vi "Actor Core.vi"(8 "error in":errorcluster, 11 "CS++DCPwrGui.lvclass":refnum<class "CS++DCPwrGui.lvclass">) -> (0 "error out":errorcluster, 3 "Actor out":refnum<class "Actor.lvclass">)   [LabVIEW 2013, in "CS++DCPwrGui.lvlib" / "CS++DCPwrGui.lvclass"]
doc: "(<B>Filename</B>: Actor Framework.lvlib:Actor.lvclass:Actor Core.vi)\n\nReceives messages to the actor, reacts to them, and initiates any error handling that may shut the actor down.\n\nDescendant classes may override this VI to append parallel tasks for the actor to complete while it handles messages. Overrides use the Call Parent Method node."
uses:
  CS++DCPwrGui.lvclass
  <vilib>/ActorFramework/Actor/Actor.lvclass
  Core/Classes/CS++ProcessVariables/ProcessVariable/PV.lvclass
  Core/Actors/CS++SVMonitor/CS++SVMonitor.lvclass
  Core/Actors/CS++BaseActor/CS++BaseActor.lvclass/CS++BaseActor.ctl
  <vilib>/ActorFramework/Actor/Actor.lvclass/Actor.ctl
  <vilib>/ActorFramework/Message Enqueuer/Message Enqueuer.lvclass/Message Enqueuer.ctl
  Core/Actors/CS++DeviceGUIActor/CS++DeviceGUIActor.lvclass/CS++DeviceGUIActor.ctl
  Core/Classes/CS++BaseClasses/Factory/CS++Factory.lvclass
  Core/Actors/CS++PVMonitor/CS++PVMonitor.lvclass/CS++PVMonitor.ctl
  Core/Actors/CS++GUIActor/CS++GUIActor.lvclass/CS++GUIActor.ctl
  CS++DMMGui Messages/UpdatePV/UpdatePV.lvclass
  Core/Actors/CS++PVMonitor Messages/Register PVs Msg/Register PVs Msg.lvclass/Register PVs Msg.ctl
  CS++DCPwrGui.lvclass/CS++DCPwrGui.ctl
  Core/Actors/CS++DeviceGUIActor/CS++DeviceGUIActor.lvclass
  Core/Classes/CS++ProcessVariables/ProcessVariable/PV.lvclass/PV.ctl
  Core/Actors/CS++DeviceGUIActor/Read Resource Name.vi
  Core/Actors/CS++DeviceGUIActor/Read Driver Revision.vi
  Core/Actors/CS++DeviceGUIActor/Read Firmware Revision.vi
  Core/Actors/CS++DeviceGUIActor/Read Self-Test Result Code.vi
  Core/Actors/CS++DeviceGUIActor/Read Self-Test Result Message.vi
  Core/Classes/CS++ProcessVariables/ProcessVariable/Read Data.vi
  <vilib>/ActorFramework/Message Enqueuer/Init from Existing Queue.vi
  <vilib>/ActorFramework/Message Enqueuer/Enqueue.vi
  <vilib>/ActorFramework/Message Priority Queue/Priority Enqueue.vi
  <vilib>/ActorFramework/Message Enqueuer/Message Enqueuer.lvclass
  Core/Actors/CS++PVMonitor Messages/Register PVs Msg/Register PVs Msg.lvclass
  <vilib>/ActorFramework/Stop Msg/Stop Msg.lvclass
  Core/Actors/CS++BaseActor/CS++BaseActor.lvclass
  Core/Actors/CS++GUIActor/CS++GUIActor.lvclass
  Core/Actors/CS++PVMonitor/CS++PVMonitor.lvclass
panel:
  in  "Tab Control":enum32{"Info", "Configuration"}(tab)
  out "Actor Name":string
  out "Driver Revision":string
  out "Firmware Revision":string
  out "Self-Test Result Code":i32
  out "Self-Test Result Message":string
  out "Resource Name":string
  in  "Configuration Tab":enum32{"General", "Trigger"}(tab)
  in  "Stop Button":bool
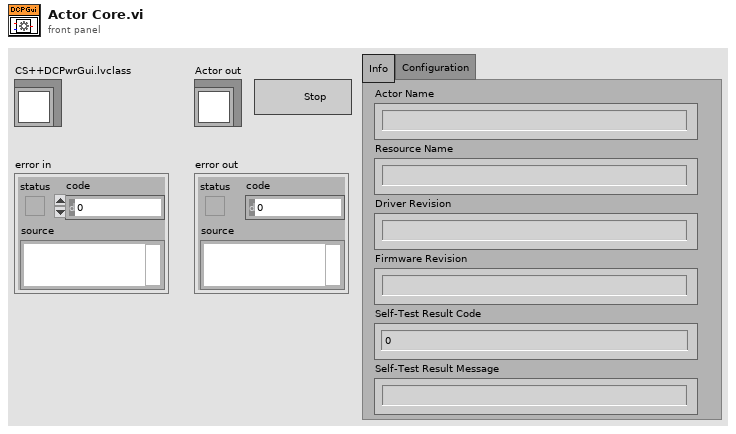
[diagram p1: front panel]
types:
  T1 = enum32{"Invalid", "Standard", "Closed", "Hidden", "Minimized", "Maximized"}
  T2 = cluster{string, "CS++DMMGui.lvlib:UpdatePV.lvclass":refnum<class "UpdatePV.lvclass">}
  T3 = cluster{"Self Enqueuer":refnum<class "Message Enqueuer.lvclass">, cluster{string, "CS++DMMGui.lvlib:UpdatePV.lvclass":refnum<class "UpdatePV.lvclass">}[]}
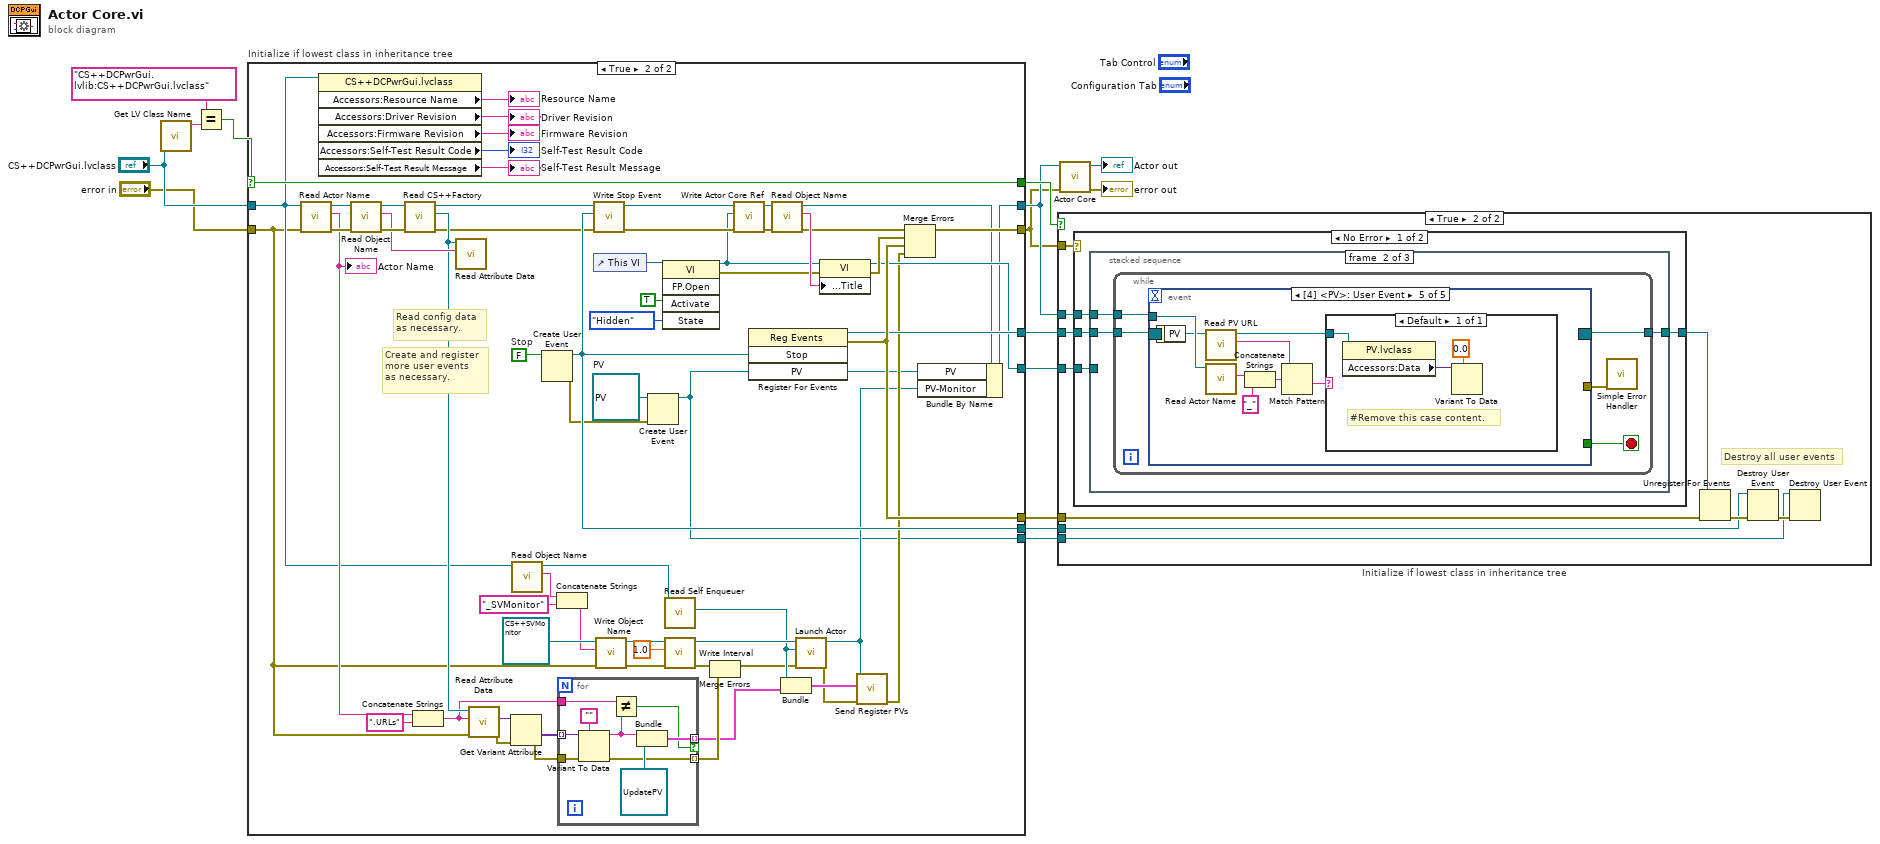
[diagram p0: block diagram]
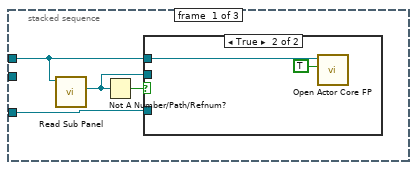
[diagram p4: hidden frame]
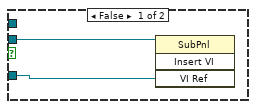
[diagram p5: hidden frame]
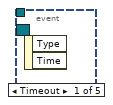
[diagram p6: hidden frame]
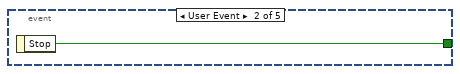
[diagram p7: hidden frame]
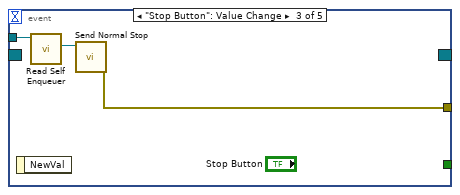
[diagram p8: hidden frame]
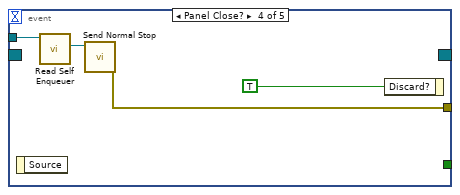
[diagram p9: hidden frame]
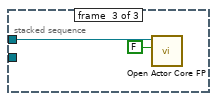
[diagram p10: hidden frame]
diagram:
  n1 = call <vilib>:"Get LV Class Name.vi"("object"="CS++DCPwrGui.lvclass") -> ("class name"=w13:string)  [unwired: 9 in, 1 out]
  n2 = Equal?(x="CS++DCPwrGui.lvlib:CS++DCPwrGui.lvclass" ("class name"), y=w13) -> (x = y?=w7:bool)
  n3 = case "Initialize if lowest class in inheritance tree" shown="True" w7 {
    selector: w7 -> [w16 w58]
    tunnel: [w17 w82] -> w2
    tunnel: "error in" -> [w17 w44]
    tunnel: [w18 w48] -> w3
    tunnel: "CS++DCPwrGui.lvclass" -> [w18 w47]
    tunnel: [_ w75] -> w11
    tunnel: [_ w74] -> w10
    tunnel: [_ w50] -> w9
    tunnel: [_ w65] -> w8
    tunnel: [w16 w58] -> w6
    tunnel: [_ w43] -> w1
    frame False {
    }
    frame True {
      w42 = refnum<class "PV.lvclass"> refnum  # PV
      w77 = FALSE  # Stop
      # "Create and register \nmore user events\nas necessary."
      # "Read config data\nas necessary."
      n4 = call "Read Actor Name.vi"("error in (no error)"=w44, "CS++GUIActor in"=w47) -> ("error out"=w68:errorcluster, "Actor Name"=w66:string, "CS++GUIActor out"=w69:refnum<class "CS++DCPwrGui.lvclass">)  [unwired: 7 in]
      "Actor Name" <- w66
      n5 = property class="CS++DCPwrGui.lvclass"(reference=w47) -> ("Accessors:Resource Name"=→"Resource Name":string, "Accessors:Driver Revision"=→"Driver Revision":string, "Accessors:Firmware Revision"=→"Firmware Revision":string, "Accessors:Self-Test Result Code"=→"Self-Test Result Code":i32, "Accessors:Self-Test Result Message"=→"Self-Test Result Message":string)  [unwired: 1 in, 2 out]
      n6 = call "Read Object Name.vi"("error in (no error)"=w68, "CS++BaseActor in"=w69) -> ("error out"=w71:errorcluster, "Object Name"=w70:string, "CS++BaseActor out"=w72:refnum<class "CS++DCPwrGui.lvclass">)  [unwired: 7 in]
      n7 = call "Read CS++Factory.vi"("error in (no error)"=w71, "CS++BaseActor in"=w72) -> ("error out"=w64:errorcluster, "CS++Factory"=w67:refnum<class "CS++Factory.lvclass">, "CS++BaseActor out"=w57:refnum<class "CS++DCPwrGui.lvclass">)  [unwired: 7 in]
      n8 = Concatenate Strings(w66, ".URLs" ("string")) -> (w23:string)
      n9 = call-dynamic "Read Attribute Data.vi"("Object Name"=w70, "CS++Factory in"=w67) -> ()  [unwired: 7 in, 3 out]
      n10 = call-dynamic "Read Attribute Data.vi"("error in (no error)"=w44, "Object Name"=w23, "CS++Factory in"=w67) -> ("error out"=w24:errorcluster, "Attribute Data"=w25:variant)  [unwired: 6 in, 1 out]
      n11 = Get Variant Attribute(Variant=w25, error in=w24) -> (values=w26:variant[], error out=w27:errorcluster)  [unwired: 2 in, 2 out]
      n12 = call "Read Object Name.vi"("CS++BaseActor in"=w47) -> ("Object Name"=w33:string, "CS++BaseActor out"=w32:refnum<class "CS++DCPwrGui.lvclass">)  [unwired: 8 in, 1 out]
      n13 = Create User Event(user event datatype=w77) -> (user event=w65:refnum<user-event>, error out=w41:errorcluster)  [unwired: 1 in]
      n14 = Concatenate Strings(w33, "_SVMonitor" ("Object Name")) -> (w37:string)
      n15 = for {
        tunnel: [w91] -> w19 mode=indexing if=w87
        tunnel: w26 -> [w90] mode=indexing
        tunnel: w27 -> [w89]
        tunnel: w23 -> [w88]
        tunnel: [w83] -> w20 mode=indexing
        n16 = Variant To Data(error in=w89, type="", Variant=w90) -> (data=w84:string, error out=w83:errorcluster)
        n17 = Not Equal?(x=w88, y=w84) -> (x != y?=w87:bool)
        n18 = Bundle(w84, "CS++DMMGui.lvlib:UpdatePV.lvclass"=refnum<class "UpdatePV.lvclass"> refnum) -> (w91:T2)  [unwired: 1 in]
      }
      n19 = call "Write Stop Event.vi"("error in (no error)"=w64, "Stop"=w65, "CS++GUIActor in"=w57) -> ("error out"=w62:errorcluster, "CS++GUIActor out"=w63:refnum<class "CS++DCPwrGui.lvclass">)  [unwired: 7 in]
      n20 = control-ref of="This VI"() -> (w81:refnum<vi>)
      n21 = call "Write Object Name.vi"("error in (no error)"=w44, "Object Name"=w37, "CS++BaseActor in"=refnum<class "CS++SVMonitor.lvclass"> refnum ("CS++SVMonitor.lvlib:CS++SVMonitor.lvclass")) -> ("error out"=w40:errorcluster, "CS++BaseActor out"=w38:refnum<class "CS++SVMonitor.lvclass">)  [unwired: 7 in]
      n22 = Create User Event(user event datatype=w42, error in=w41) -> (user event=w43:refnum<user-event>)  [unwired: 1 out]
      n23 = invoke class="VI" method="FP.Open"(reference=w81, "Activate"=TRUE ("Activate?"), "State"=T1."Hidden") -> (reference out=w51:refnum<vi>, error out=w73:errorcluster)  [unwired: 2 in, 3 out]
      n24 = call <vilib>:"Read Self Enqueuer.vi"("Actor"=w32) -> ("Self Enqueuer"=w31:refnum<class "Message Enqueuer.lvclass">)  [unwired: 10 in]
      n25 = call "Write Interval.vi"("error in (no error)"=w40, "Interval"=dbl[unit] 1.0, "CS++PVMonitor in"=w38) -> ("error out"=w22:errorcluster, "CS++PVMonitor out"=w36:refnum<class "CS++SVMonitor.lvclass">)  [unwired: 7 in]
      n26 = Merge Errors(w22, w20) -> (w21:errorcluster)
      n27 = call "Write Actor Core Ref.vi"("error in (no error)"=w62, "Actor Core Ref"=w51, "CS++BaseActor in"=w63) -> ("error out"=w61:errorcluster, "CS++BaseActor out"=w60:refnum<class "CS++DCPwrGui.lvclass">)  [unwired: 7 in]
      n28 = register-events(w65, w43) -> (reference out=w74:refnum<event-registration>, error out=w75:errorcluster)  [unwired: 2 in]
      n29 = call "Read Object Name.vi"("error in (no error)"=w61, "CS++BaseActor in"=w60) -> ("error out"=w59:errorcluster, "Object Name"=w78:string, "CS++BaseActor out"=w49:refnum<class "CS++DCPwrGui.lvclass">)  [unwired: 7 in]
      n30 = Bundle("Self Enqueuer"=w31, w19) -> (w30:T3)  [unwired: 1 in]
      n31 = call <vilib>:"Launch Actor.vi"("error in (no error)"=w21, "Actor-to-Caller Enqueuer"=w31, "Actor"=w36) -> ("error out"=w29:errorcluster, "Caller-To-Actor Enqueuer"=w45:refnum<class "Message Enqueuer.lvclass">)  [unwired: 7 in]
      n32 = property class="VI"(reference=w51, error in=w73, "Front Panel.Title"=w78) -> (reference out=w50:refnum<vi>, error out=w76:errorcluster)
      n33 = call "Send Register PVs.vi"("error in (no error)"=w29, "Register Info"=w30, "Message Enqueuer"=w45) -> ("error out"=w46:errorcluster)  [unwired: 7 in, 1 out]
      n34 = Merge Errors(w59, w76, w75, w46) -> (w82:errorcluster)
      n35 = Bundle By Name(cluster=w49, "PV"=w43, "PV-Monitor"=w45) -> (w48:refnum<class "CS++DCPwrGui.lvclass">)
    }
  }
  n36 = case "Initialize if lowest class in inheritance tree" shown="True" w6 {
    tunnel: w2 -> [_ w101]
    tunnel: w3 -> [_ w100]
    tunnel: w11 -> [_ w98]
    tunnel: w10 -> [_ w97]
    tunnel: w9 -> [_ w95]
    tunnel: w8 -> [_ w94]
    tunnel: w1 -> [_ w92]
    frame False {
    }
    frame True {
      # "Destroy all user events"
      n37 = case shown="No Error" w101 {
        tunnel: w100 -> [w105 _]
        tunnel: w97 -> [w104 w143]
        tunnel: [w103 w143] -> w96
        tunnel: w95 -> [w102 _]
        frame No Error {
          n38 = stacked-sequence {
            tunnel: w105 -> [w107 w115 w142]
            tunnel: w104 -> [_ w116 _]
            tunnel: [_ w114 _] -> w103
            tunnel: w102 -> [w108 _ _]
            frame #0 {
              n39 = call "Read Sub Panel.vi"("CS++GUIActor in"=w107) -> ("Sub Panel"=w106:refnum<vi>)  [unwired: 8 in, 2 out]
              n40 = Not A Number/Path/Refnum?(number/path/refnum=w106) -> (NaN/Path/Refnum?=w109:bool)
              n41 = case shown="True" w109 {
                tunnel: w107 -> [_ w113]
                tunnel: w106 -> [w111 _]
                tunnel: w108 -> [w110 _]
                frame False {
                  n42 = invoke class="SubPnl" method="Insert VI"(reference=w111, "VI Ref"=w110) -> ()  [unwired: 2 in, 4 out]
                }
                frame True {
                  n43 = call "Open Actor Core FP.vi"("Open FP (F)"=TRUE, "CS++BaseActor in"=w113) -> ()  [unwired: 8 in, 2 out]
                }
              }
            }
            frame #1 {
              n44 = while {
                tunnel: w116 -> [w121]
                tunnel: w115 -> [w120]
                tunnel: [w118] -> w114
                stop <- w119 stop-if-true
                n45 = event shown="[4] <PV>: User Event" {
                  selector: w121 -> [_ _ _ _ _]
                  dyn-events: [_ _ _ _ _] -> w118
                  timeout: _ -> [_ _ _ _ _]
                  tunnel: w120 -> [_ _ w125 w127 w134]
                  tunnel: [_ w122 _ _ _] -> w119
                  tunnel: [_ _ w123 w126 _] -> w117
                  event Timeout {
                    n46 = event-data() -> ()  [unwired: 1 in, 2 out]
                  }
                  event User Event {
                    n47 = event-data() -> ("Stop"=w122:bool)  [unwired: 1 in]
                  }
                  event "Stop Button": Value Change {
                    n48 = event-data() -> ()  [unwired: 1 in, 1 out]
                    n49 = call <vilib>:"Read Self Enqueuer.vi"("Actor"=w125) -> ("Self Enqueuer"=w124:refnum<class "Message Enqueuer.lvclass">)  [unwired: 10 in]
                    n50 = call <vilib>:"Send Normal Stop.vi"("Message Enqueuer"=w124) -> ("error out"=w123:errorcluster)  [unwired: 10 in]
                  }
                  event Panel Close? {
                    n51 = event-data() -> ()  [unwired: 1 in, 1 out]
                    n52 = call <vilib>:"Read Self Enqueuer.vi"("Actor"=w127) -> ("Self Enqueuer"=w128:refnum<class "Message Enqueuer.lvclass">)  [unwired: 10 in]
                    n53 = call <vilib>:"Send Normal Stop.vi"("Message Enqueuer"=w128) -> ("error out"=w126:errorcluster)  [unwired: 10 in]
                    n54 = event-data("Discard?"=TRUE) -> ()  [unwired: 1 in, 1 out]
                  }
                  event User Event {
                    n55 = event-data() -> ("PV"=w133:refnum<class "PV.lvclass">)  [unwired: 1 in]
                    n56 = call "Read PV URL.vi"("PV in"=w133) -> ("PV URL"=w132:string, "PV out"=w130:refnum<class "PV.lvclass">)  [unwired: 8 in, 1 out]
                    n57 = call "Read Actor Name.vi"("CS++GUIActor in"=w134) -> ("Actor Name"=w136:string)  [unwired: 8 in, 2 out]
                    n58 = Concatenate Strings(w136, "_" ("string")) -> (w137:string)
                    n59 = Match Pattern(string=w132, regular expression=w137) -> (after substring=w131:string)  [unwired: 1 in, 3 out]
                    n60 = case shown="Default" w131 {
                      tunnel: w130 -> [w138]
                      frame Default {
                        # "#Remove this case content."
                        n61 = property class="PV.lvclass"(reference=w138) -> ("Accessors:Data"=w139:variant)  [unwired: 1 in, 2 out]
                        n62 = Variant To Data(type=0.0, Variant=w139) -> ()  [unwired: 1 in, 2 out]
                      }
                    }
                  }
                }
                n63 = call <vilib>:"Simple Error Handler.vi"("error in (no error)"=w117) -> ()  [unwired: 4 in, 5 out]
              }
            }
            frame #2 {
              n64 = call "Open Actor Core FP.vi"("Open FP (F)"=FALSE, "CS++BaseActor in"=w142) -> ()  [unwired: 8 in, 2 out]
            }
          }
        }
        frame Error {
        }
      }
      n65 = Unregister For Events(event registration refnum=w96, error in=w98) -> (error out=w99:errorcluster)
      n66 = Destroy User Event(user event=w94, error in=w99) -> (error out=w93:errorcluster)
      n67 = Destroy User Event(user event=w92, error in=w93) -> ()  [unwired: 1 out]
    }
  }
  n68 = call-parent "Actor Core.vi"("error in"=w2, "CS++DeviceGUIActor.lvclass"=w3) -> ("error out"=→"error out":errorcluster, "Actor out"=→"Actor out":refnum<class "Actor.lvclass">)  [unwired: 8 in]
